vi "Capture from UV Camera.vi"(8 "error in":errorcluster, 11 "Image number in":i32) -> (0 "error out":errorcluster, 2 "Image Out":T1(plugin-control), 3 "Image number out":i32)   [LabVIEW 2013]
doc: "This sub-VI captures an image using the UV camera and saves the acquired image to a file in the\n[Application]/Data directory."
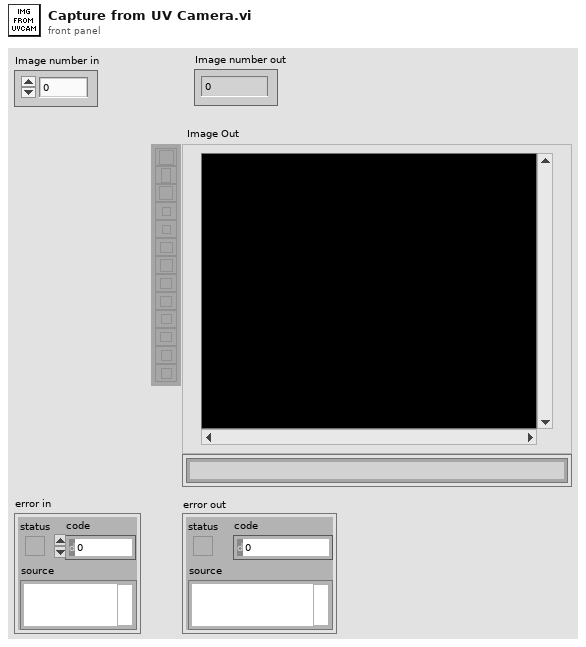
[diagram p1: front panel]
types:
  T1 = typedef "IMAQ Image.ctl" = refnum<image>
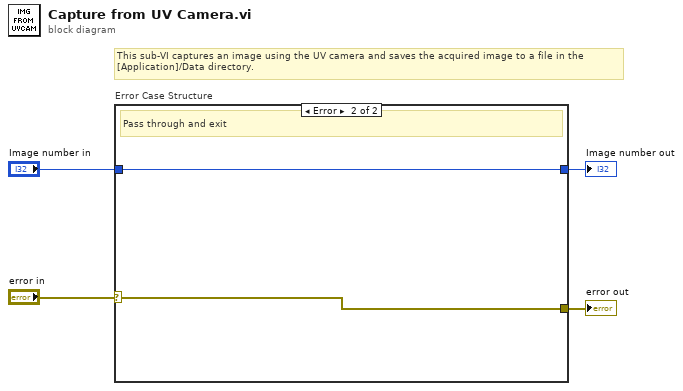
[diagram p0: block diagram]
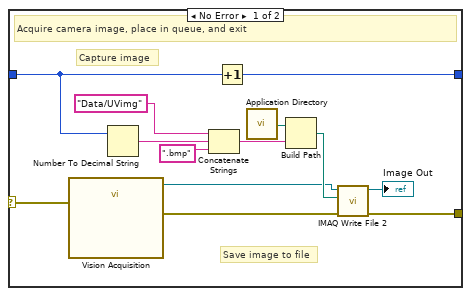
[diagram p2: hidden frame]
diagram:
  # "This sub-VI captures an image using the UV camera and saves the acquired image to a file in the\n[Application]/Data directory."
  n1 = case "Error Case Structure" shown="Error" "error in" {
    selector: "error in" -> [w17 w19]
    tunnel: [w8 w19] -> w4
    tunnel: "Image number in" -> [w5 w18]
    tunnel: [w16 w18] -> w1
    frame No Error {
      # "Save image to file"
      # "Capture image"
      # "Acquire camera image, place in queue, and exit"
      n2 = call "Vision Acquisition"("error in"=w17) -> ("Image Out"=w7:T1, "error out"=w9:errorcluster)  [unwired: 25 in]
      n3 = Number To Decimal String(number=w5) -> (decimal integer string=w12:string)  [unwired: 1 in]
      n4 = Concatenate Strings("Data/UVimg" ("name or relative path"), w12, ".bmp" ("string")) -> (w14:string)
      n5 = Increment(x=w5) -> (x+1=w16:i32)
      n6 = call <vilib>:"Application Directory.vi"() -> ("Application Directory"=w10:path)
      n7 = Build Path(base path=w10, name or relative path=w14) -> (appended path=w15:path)
      n8 = call-poly "IMAQ Write File 2"("error in (no error)"=w9, "File Path"=w15, "Image"=w7) -> ("error out"=w8:errorcluster, "Image Out (duplicate)"=→"Image Out":T1)  [unwired: 7 in]
    }
    frame Error {
      # "Pass through and exit"
    }
  }
  "error out" <- w4
  "Image number out" <- w1
